vi "BypassAndLogErrors -- V2.vi"(6 "Log Error ?":bool=TRUE, 7 "Bypass Errors":bool, 8 "error in (no error)":errorcluster, 11 "Log File Path":path) -> (0 "error out":errorcluster)   [LabVIEW 2015]
panel:
  out "resulting string":string
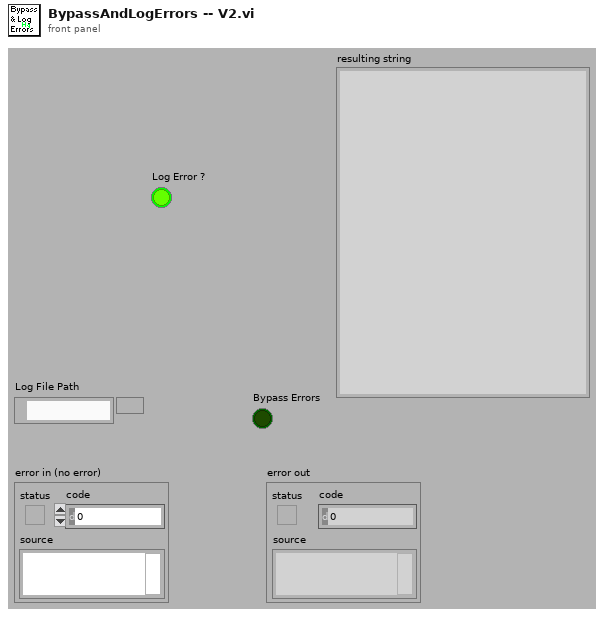
[diagram p1: front panel]
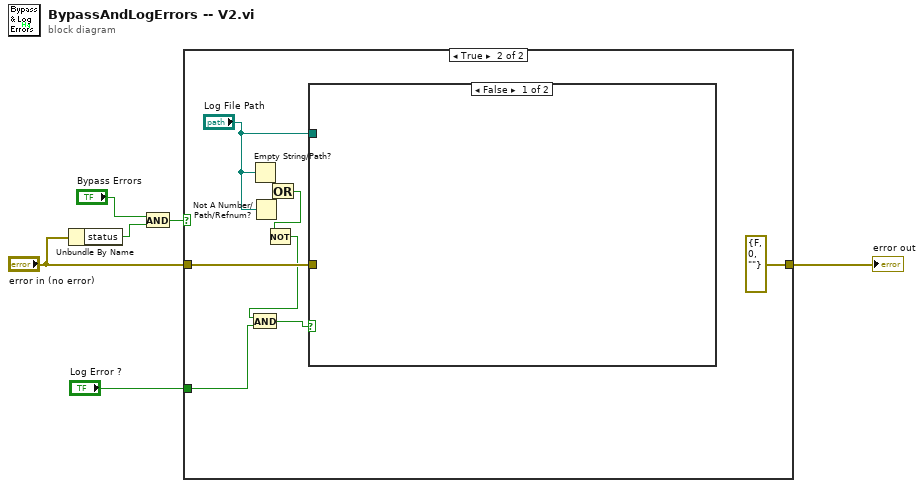
[diagram p0: block diagram]
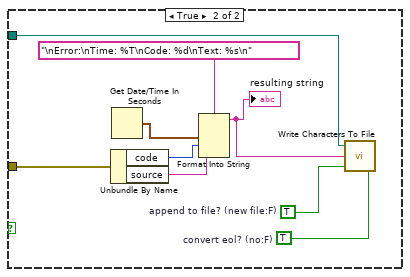
[diagram p3: hidden frame]
diagram:
  n1 = Unbundle By Name("error in (no error)") -> ("status"=w3:bool)
  n2 = And(x="Bypass Errors", y=w3) -> (x .and. y?=w2:bool)
  n3 = case shown="True" w2 {
    tunnel: [w7 errorcluster {"status"=FALSE, "code"=0, "source"=""} ("error in (no error)")] -> w6
    tunnel: "error in (no error)" -> [w7 w15]
    tunnel: "Log Error ?" -> [_ w12]
    frame False {
    }
    frame True {
      n4 = Empty String/Path?(string/path="Log File Path") -> (empty?=w13:bool)
      n5 = Not A Number/Path/Refnum?(number/path/refnum="Log File Path") -> (NaN/Path/Refnum?=w11:bool)
      n6 = Or(x=w13, y=w11) -> (x .or. y?=w9:bool)
      n7 = Not(x=w9) -> (.not. x?=w10:bool)
      n8 = And(x=w10, y=w12) -> (x .and. y?=w8:bool)
      n9 = case shown="False" w8 {
        tunnel: w15 -> [_ w24]
        tunnel: "Log File Path" -> [_ w19]
        frame False {
        }
        frame True {
          w17 = TRUE  # convert eol? (no:F)
          w25 = TRUE  # append to file? (new file:F)
          n10 = Unbundle By Name(w24) -> ("code"=w22:i32, "source"=w21:string)
          n11 = Get Date/Time In Seconds() -> (seconds since 1Jan1904=w23:timestamp)
          n12 = Format Into String(format string="\nError:\nTime: %T\nCode: %d\nText: %s\n", w23, w22, w21) -> (resulting string=w20:string)  [unwired: 2 in, 1 out]
          "resulting string" <- w20
          n13 = call <vilib>:"Write Characters To File.vi"("convert eol? (no:F)"=w17, "append to file? (new file:F)"=w25, "character string"=w20, "file path (dialog if empty)"=w19) -> ()  [unwired: 2 out]
        }
      }
    }
  }
  "error out" <- w6
